vi "Cal_stage_to_theta.vi"(10 "file path (dialog if empty)":path) -> (3 "predicted theta":dbl)   [LabVIEW 2012]
uses:
  <vilib>/Utility/file.llb/Read From Spreadsheet File (DBL).vi
  variables/GlobalUI.vi
  <vilib>/gmath/NI_Gmath.lvlib
panel:
  out "reference table":dbl[][](array[numeric]) format="%0.3f"
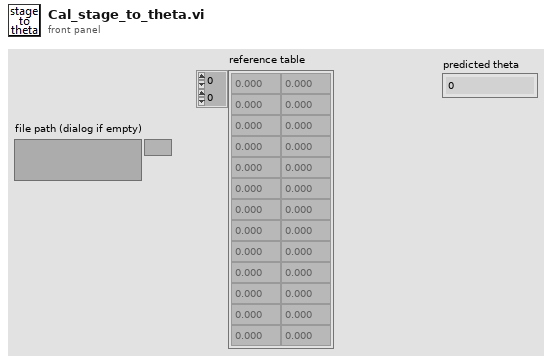
[diagram p1: front panel]
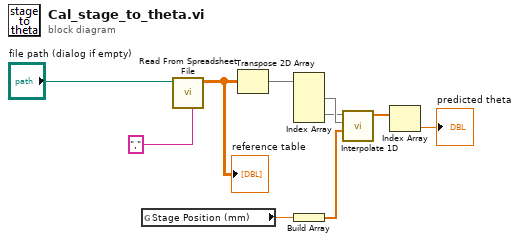
[diagram p0: block diagram]
diagram:
  n1 = global read "GlobalUI.vi" "Stage Position (mm)"() -> (w1:dbl)
  n2 = call-poly <vilib>:"Read From Spreadsheet File.vi"("delimiter (\\t)"="," ("delimiter (\\t)"), "file path (dialog if empty)"="file path (dialog if empty)") -> ("all rows"=w8:dbl[][])  [unwired: 5 in, 4 out]
  "reference table" <- w8
  n3 = Transpose 2D Array(2D array=w8) -> (transposed array=w7:dbl[][])
  n4 = Index Array(array=w7) -> (element #1=w6:dbl[], element #2=w5:dbl[])  [unwired: 4 in]
  n5 = Build Array(w1) -> (w4:dbl[])
  n6 = call <vilib>:"Interpolate 1D.vi"("xi"=w4, "X"=w6, "Y"=w5) -> ("yi"=w3:dbl[])  [unwired: 6 in, 2 out]
  n7 = Index Array(array=w3) -> (element=→"predicted theta":dbl)  [unwired: 1 in]
